vi "Linear Fit Coefficients (LS).vi"(0 "Y":dbl[](array[numeric]) format="%0.2f", 5 "X":dbl[](array[numeric]) format="%0.2f", 7 "Weight":dbl[](array[numeric]) format="%0.2f") -> (4 "slope":dbl format="%0.2f", 6 "intercept":dbl format="%0.2f", 15 "error":i32)   [LabVIEW 2017, in "NI_AALPro.lvlib"]
uses:
  NI_AALPro.lvlib
  <resource>/lvanlys.dll
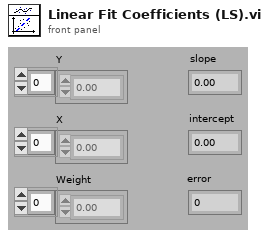
[diagram p1: front panel]
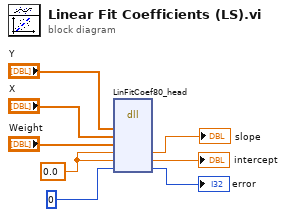
[diagram p0: block diagram]
diagram:
  w1 = 0.0
  n1 = dll-call lib="C:/Program Files (x86)/National Instruments/LabVIEW 2017/resource/lvanlys.*" fn="LinFitCoef80_head"("yH"="Y", "xH"="X", "wH"="Weight", "slope"=w1, "intercept"=w1, "dsperr"=0) -> ("slope"=→"slope":dbl, "intercept"=→"intercept":dbl, "dsperr"=→"error":i32)  [unwired: 7 in, 2 out]
